vi "Reset.vi"(8 "error in (no error)":errorcluster, 10 "Message in":refnum<class "ResetMessage.lvclass">, 11 "RSA in":refnum<class "RSA.lvclass">) -> (0 "error out":errorcluster, 3 "RSA out":refnum<class "RSA.lvclass">)   [LabVIEW 2012, in "RSA.lvclass"]
doc: "The reset method processes the command 'reset'. \n\nResets the internal state of the component (without performing a full initialisation). This could be resetting hardware, or private data to default values."
uses:
  RSA.lvclass
  <vilib>/Distrio/Murmex/ResetMessage/ResetMessage.lvclass
  <vilib>/Distrio/Murmex/Murmex/Murmex.lvclass
  RSA.lvclass/RSA.ctl
panel:
  # "This method is called when the RESET\ntrigger is sent. \n\nOverride this method when your component needs to\nrespond to this trigger. \n\nCall parent for proper implementation"
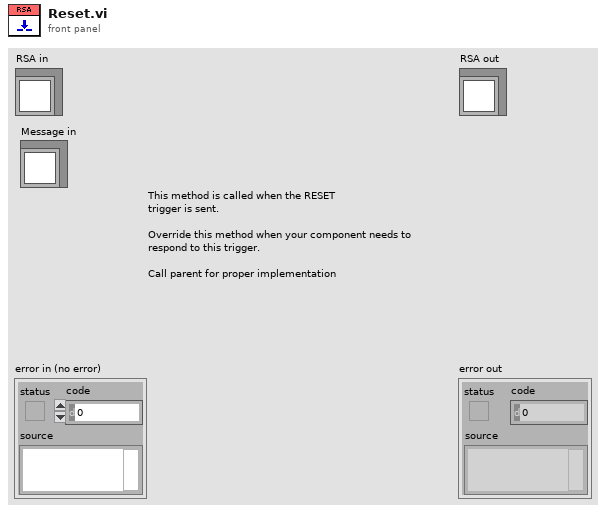
[diagram p1: front panel]
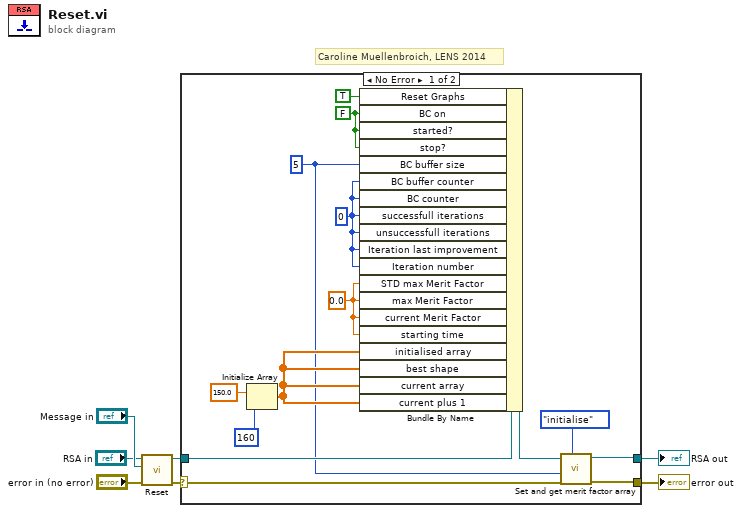
[diagram p0: block diagram]
diagram:
  # "Caroline Muellenbroich, LENS 2014"
  n1 = call-parent "Reset.vi"("error in (no error)"="error in (no error)", "Message in"="Message in", "Murmex in"="RSA in") -> ("error out"=w4:errorcluster, "Murmex out"=w2:refnum<class "RSA.lvclass">)  [unwired: 7 in]
  n2 = case shown="No Error" w4 {
    selector: w4 -> [w13 w22]
    tunnel: [w15 w22] -> w3
    tunnel: w2 -> [w14 w23]
    tunnel: [w16 w23] -> w1
    frame No Error {
      w12 = FALSE ("Run time cluster.BC on")
      w11 = 5 ("Settings Cluster.BC buffer size")
      w10 = 0 ("Run time cluster.Iteration number")
      w9 = 0.0 ("Run time cluster.current Merit Factor")
      n3 = Initialize Array(150.0 ("element"), 160 ("dimension size")) -> (w21:dbl[])
      n4 = Bundle By Name(cluster=w14, "Reset Graphs"=TRUE ("Run time cluster.Reset Graphs"), "BC on"=w12, "started?"=w12, "stop?"=w12, "BC buffer size"=w11, "BC buffer counter"=w10, "BC counter"=w10, "successfull iterations"=w10, "unsuccessfull iterations"=w10, "Iteration last improvement"=w10, "Iteration number"=w10, "STD max Merit Factor"=w9, "max Merit Factor"=w9, "current Merit Factor"=w9, "starting time"=w9, "initialised array"=w21, "best shape"=w21, "current array"=w21, "current plus 1"=w21) -> (w17:refnum<class "RSA.lvclass">)
      n5 = call "Set and get merit factor array.vi"("action"=enum16{"set", "get", "initialise"}."initialise", "error in (no error)"=w13, "array size"=w11, "RSA in"=w17) -> ("error out"=w15:errorcluster, "RSA out"=w16:refnum<class "RSA.lvclass">)  [unwired: 4 in, 2 out]
    }
    frame Error {
    }
  }
  "error out" <- w3
  "RSA out" <- w1
